vi "GetDataGroupStatus.vi"(8 "error in":errorcluster, 10 "status":variant, 11 "data group":string) -> (0 "error out":errorcluster, 3 "CurrentOpState":i32)   [LabVIEW 2017, in "OpState.lvlib"]
uses:
  <vilib>/addons/InsightCM/Devices/Shared/Common/OpState/OpState.lvlib
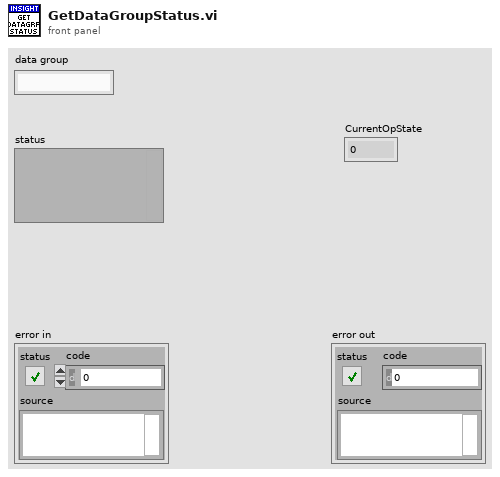
[diagram p1: front panel]
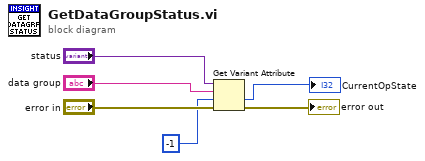
[diagram p0: block diagram]
diagram:
  n1 = Get Variant Attribute(Variant="status", name="data group", default value (empty Variant)=-1 ("CurrentOpState"), error in="error in") -> (value=→"CurrentOpState":i32, error out=→"error out":errorcluster)  [unwired: 2 out]
